vi "Test Script.vi"() -> ()   [LabVIEW 2016, in "User Interface.lvlib"]
uses:
  User Interface.lvlib
panel:
  in  "Test Description":T1(array[cluster])
  out "Time":string="Sat  8/3/2019  8:10:44 PM"
  in  "Exit?":bool
  in  "Exit":bool
  out "error out":errorcluster
  in  "error in (no error)":errorcluster
  # "Test Script"
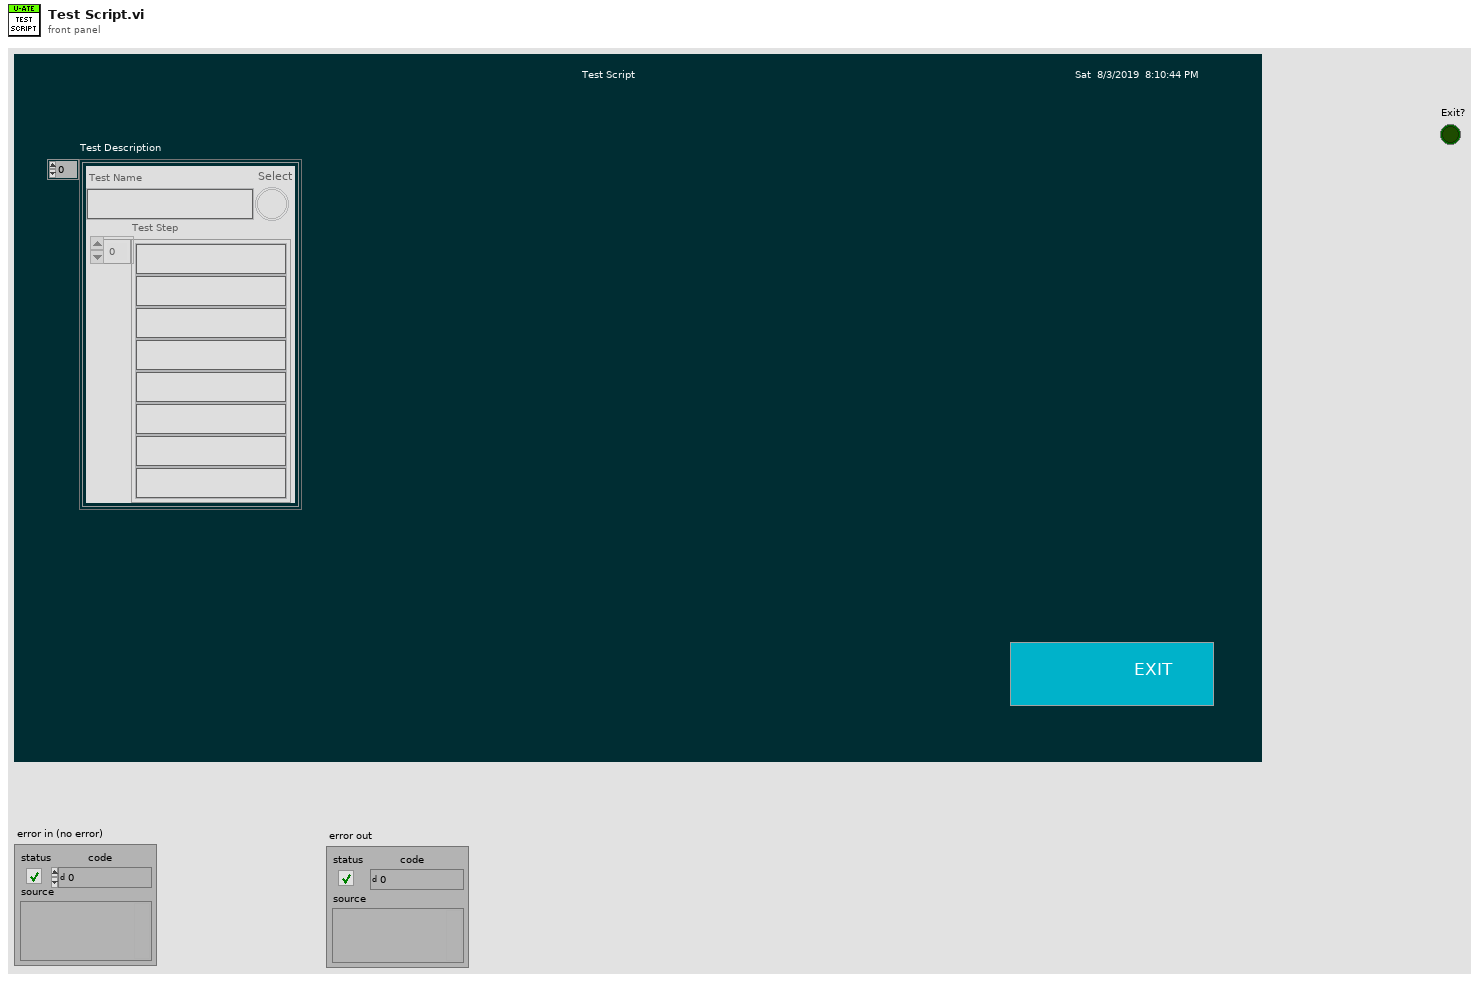
[diagram p1: front panel]
types:
  T1 = cluster{"Select":bool, "Test Name":string, "Test Step":string[]}[]
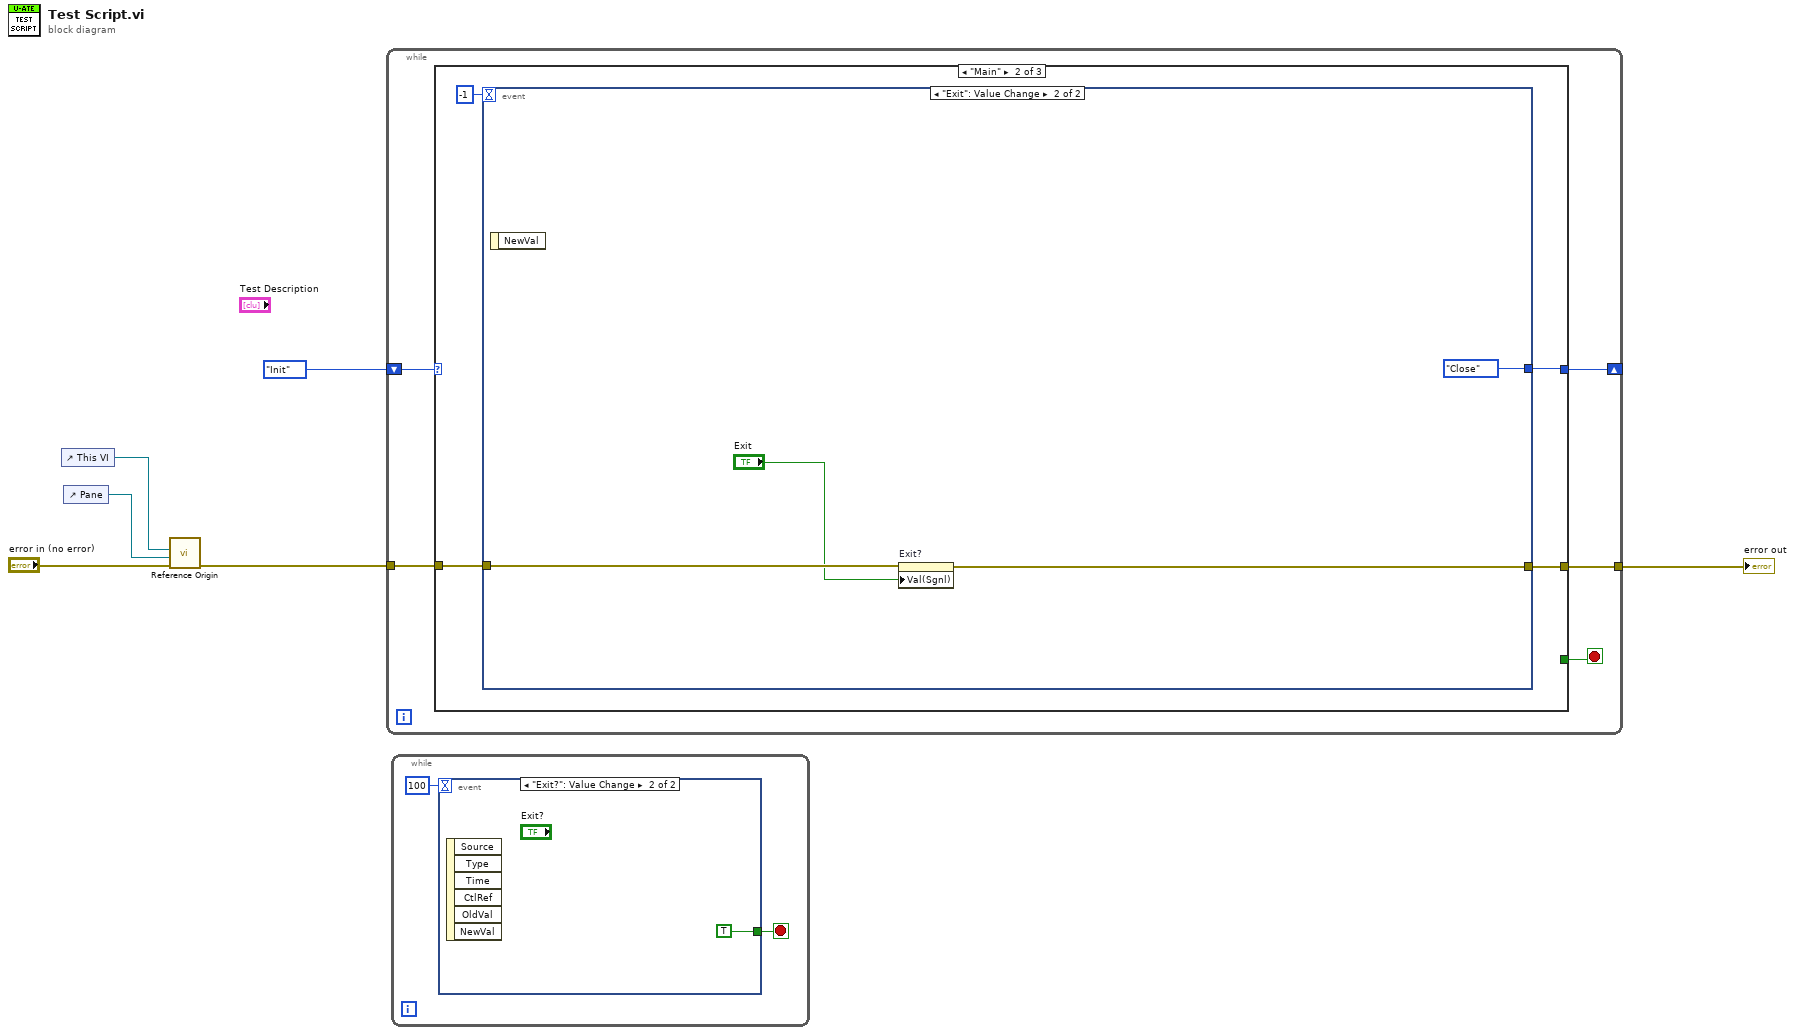
[diagram p0: block diagram]
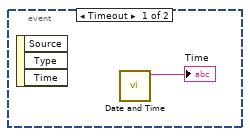
[diagram p2: hidden frame]
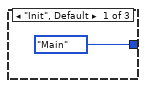
[diagram p3: hidden frame]
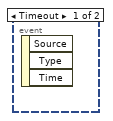
[diagram p4: hidden frame]
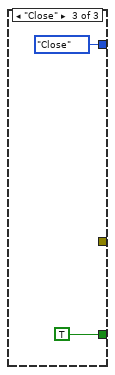
[diagram p5: hidden frame]
diagram:
  n1 = control-ref of="This VI"() -> (w5:refnum<vi>)
  n2 = control-ref of="Pane"() -> (w4:refnum<vi>)
  n3 = call "Reference Origin.vi"("error in (no error)"="error in (no error)", "Pane"=w4, "This VI"=w5) -> ("error out"=w3:errorcluster)  [unwired: 8 in]
  n4 = while {
    tunnel: w3 -> [w11]
    shift-right: [w9] -> _
    shift-left: enum16{"Init", "Main", "Close"}."Init" -> [w10]
    tunnel: [w8] -> w1
    stop <- w7 stop-if-true
    n5 = case shown="\"Main\"" w10 {
      tunnel: w11 -> [_ w16 _]
      tunnel: [enum16{"Init", "Main", "Close"}."Main" w13 enum16{"Init", "Main", "Close"}."Close"] -> w9
      tunnel: [_ w14 _] -> w8
      tunnel: [_ _ TRUE] -> w7
      frame "Init", Default {
      }
      frame "Main" {
        n6 = event shown="[1] \"Exit\": Value Change" {
          selector: _ -> [_ _]
          dyn-events: _ -> [_ _]
          timeout: -1 -> [_ _]
          tunnel: w16 -> [_ w20]
          tunnel: [_ w18] -> w14
          tunnel: [_ enum16{"Init", "Main", "Close"}."Close"] -> w13
          event Timeout {
            n7 = event-data() -> ()  [unwired: 1 in, 3 out]
          }
          event "Exit": Value Change {
            n8 = event-data() -> ()  [unwired: 1 in, 1 out]
            n9 = property on="Exit?" class="Bool (strict)"(error in=w20, "Val(Sgnl)"="Exit") -> (error out=w18:errorcluster)  [unwired: 1 in, 1 out]
          }
        }
      }
      frame "Close" {
      }
    }
  }
  "error out" <- w1
  n10 = while {
    stop <- w23 stop-if-true
    n11 = event shown="[1] \"Exit?\": Value Change" {
      selector: _ -> [_ _]
      dyn-events: _ -> [_ _]
      timeout: 100 -> [_ _]
      tunnel: [_ TRUE] -> w23
      event Timeout {
        n12 = event-data() -> ()  [unwired: 1 in, 3 out]
        n13 = call "Date and Time.vi"() -> ("Current Time"=→"Time":string)  [unwired: 11 in]
      }
      event "Exit?": Value Change {
        n14 = event-data() -> ()  [unwired: 1 in, 6 out]
      }
    }
  }
